vi "TDMS Read Channel Custom Fields.vi"(4 "MN":string, 5 "System or ALL Combined Fields":T1[](array[typedef]), 6 "SN":string, 7 "Group Name":string, 8 "error in (no error)":errorcluster, 9 "Channel":string, 10 "Custom Field Records to Search":string[](array[string]), 11 "tdms file ref":refnum<k34>) -> (0 "error out":errorcluster, 2 "Custom Fields":T1[](array[typedef]), 3 "tdms file ref":refnum<k34>)   [LabVIEW 2011]
uses:
  typedefs/Field Record.ctl
  typedefs/Field DataTypes.ctl
  typedefs/Field NextItem.ctl
panel:
  out "x-y 2":u32
  out "x-y":u32
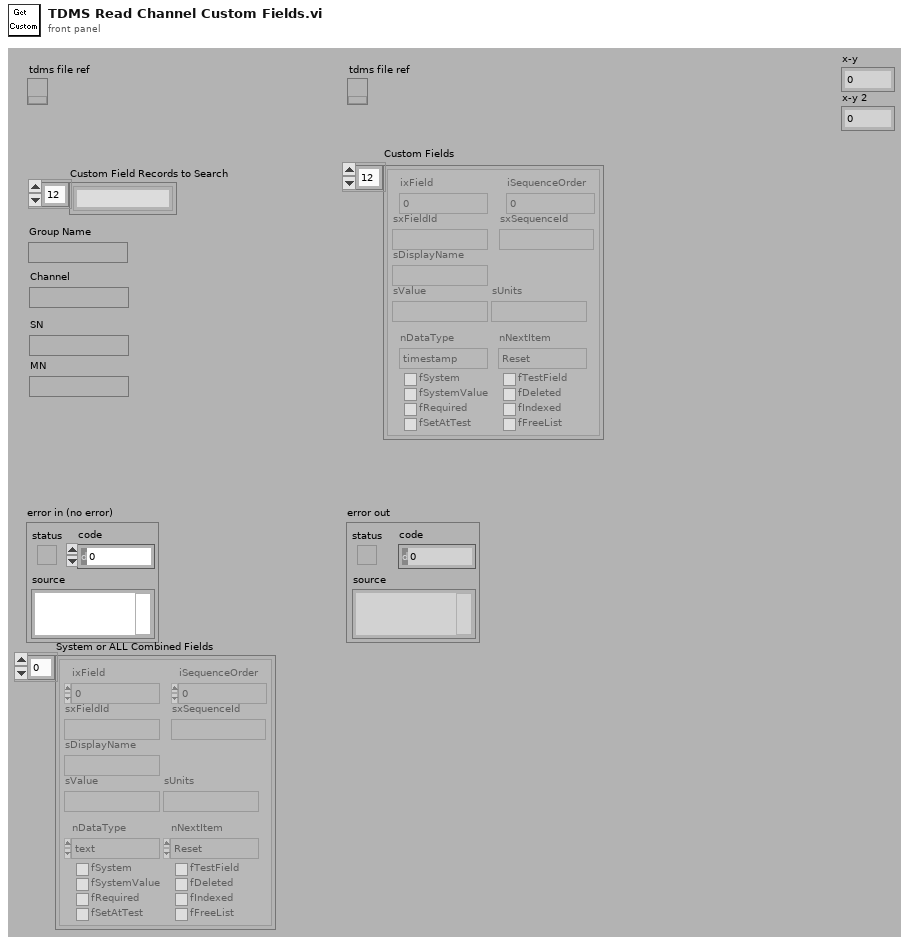
[diagram p1: front panel]
types:
  T1 = typedef "Field Record.ctl" = cluster{"ixField":i32, "iSequenceOrder":i32, "sxFieldId":string, "sxSequenceId":string, "sDisplayName":string, "sValue":string, "sUnits":string, "nDataType":T2, "nNextItem":T3, "fSystem":bool, "fSystemValue":bool, "fRequired":bool, "fSetAtTest":bool, "fTestField":bool, "fDeleted":bool, "fIndexed":bool, "fFreeList":bool}
  T2 = typedef "Field DataTypes.ctl" = enum32{"text", "numeric", "list", "timestamp", "boolean"}
  T3 = typedef "Field NextItem.ctl" = enum32{"Reset", "Retain", "Auto-Increment"}
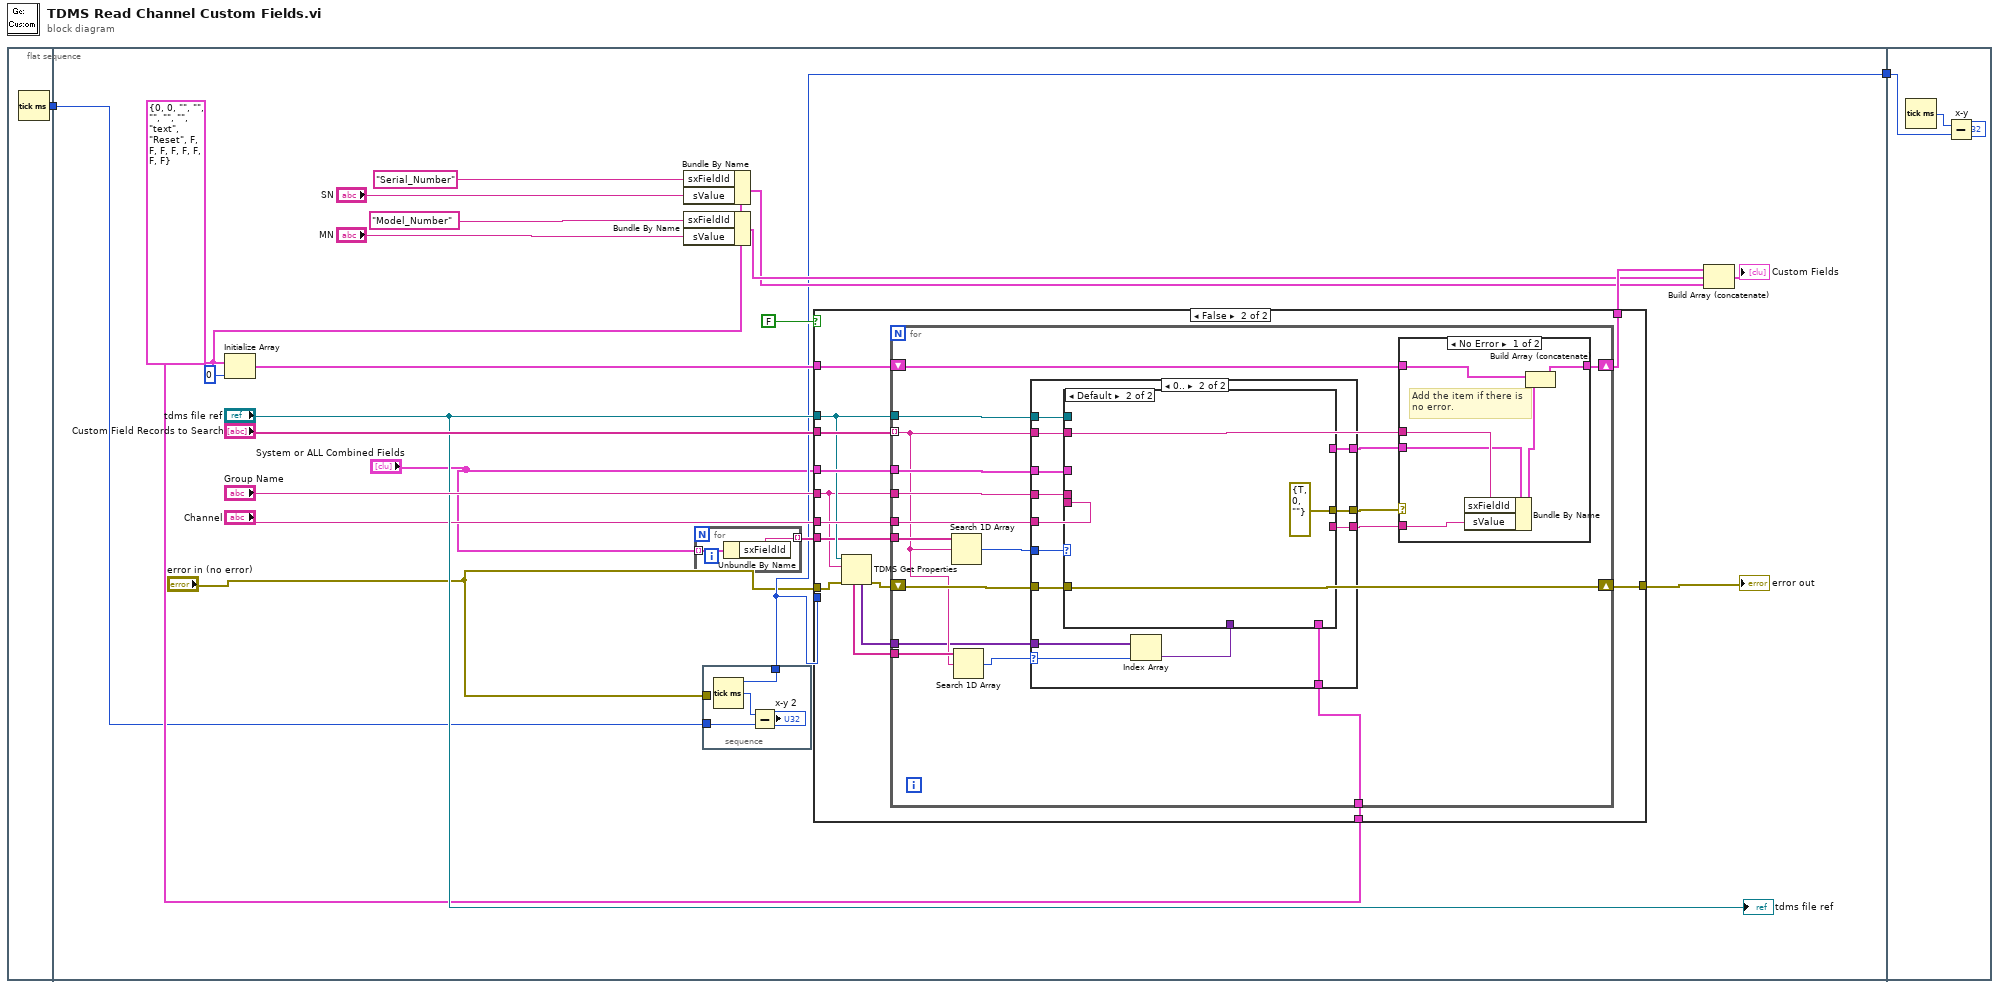
[diagram p0: block diagram]
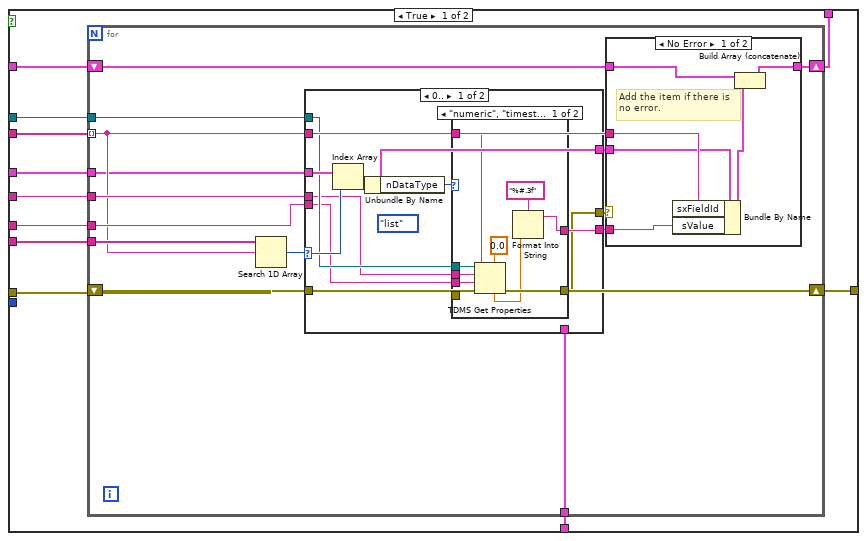
[diagram p2: hidden frame]
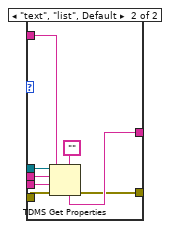
[diagram p3: hidden frame]
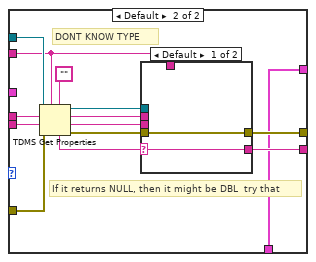
[diagram p4: hidden frame]
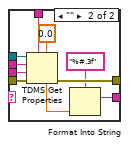
[diagram p5: hidden frame]
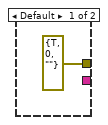
[diagram p7: hidden frame]
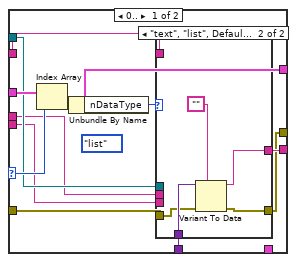
[diagram p8: hidden frame]
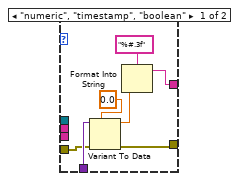
[diagram p9: hidden frame]
diagram:
  n1 = flat-sequence {
    tunnel: [w3] -> w1
    tunnel: [w7] -> w2
    tunnel: w1 -> [w6]
    tunnel: w2 -> [w197]
    frame #0 {
      n2 = Tick Count (ms)() -> (millisecond timer value=w3:u32)
    }
    frame #1 {
      w17 = T1 {"ixField"=0, "iSequenceOrder"=0, "sxFieldId"="", "sxSequenceId"="", "sDisplayName"="", "sValue"="", "sUnits"="", "nDataType"=enum."text", "nNextItem"=enum."Reset", "fSystem"=FALSE, "fSystemValue"=FALSE, "fRequired"=FALSE, "fSetAtTest"=FALSE, "fTestField"=FALSE, "fDeleted"=FALSE, "fIndexed"=FALSE, "fFreeList"=FALSE} ("Field Record")
      n3 = Initialize Array(w17, 0 ("dimension size")) -> (w25:T1[])
      n4 = Bundle By Name(cluster=w17, "sxFieldId"="Serial_Number", "sValue"="SN") -> (w9:T1)
      n5 = Bundle By Name(cluster=w17, "sxFieldId"="Model_Number", "sValue"="MN") -> (w10:T1)
      n6 = for {
        tunnel: "System or ALL Combined Fields" -> [w195] mode=indexing
        tunnel: [w194] -> w18 mode=indexing
        n7 = Unbundle By Name(w195) -> ("sxFieldId"=w194:string)
      }
      n8 = stacked-sequence {
        tunnel: "error in (no error)" -> [_]
        tunnel: [w28] -> w7
        tunnel: w6 -> [w27]
        frame #0 {
          n9 = Tick Count (ms)() -> (millisecond timer value=w28:u32)
          n10 = Subtract(x=w28, y=w27) -> (x-y=→"x-y 2":u32)
        }
      }
      n11 = case shown="False" FALSE {
        tunnel: w25 -> [w39 w129]
        tunnel: [w38 w128] -> w23
        tunnel: "Custom Field Records to Search" -> [w37 w127]
        tunnel: "Group Name" -> [w36 w118]
        tunnel: "tdms file ref" -> [w35 w120]
        tunnel: "Channel" -> [w34 w126]
        tunnel: "error in (no error)" -> [w33 w122]
        tunnel: w18 -> [w32 w119]
        tunnel: "System or ALL Combined Fields" -> [w31 w125]
        tunnel: w17 -> [w30 w124]
        tunnel: [w29 w123] -> w11
        tunnel: w7 -> [_ _]
        frame True {
          n12 = for {
            shift-right: [w51] -> w38
            shift-left: w33 -> [w51]
            shift-right: [w52] -> w29
            shift-left: w39 -> [w53]
            tunnel: w35 -> [w48]
            tunnel: w37 -> [w44] mode=indexing
            tunnel: w36 -> [w49]
            tunnel: w30 -> [w40]
            tunnel: w34 -> [w46]
            tunnel: w32 -> [w45]
            tunnel: w31 -> [w42]
            n13 = Search 1D Array(1D array=w45, element=w44) -> (index of element=w43:i32)  [unwired: 1 out]
            n14 = case shown="0.." w43 {
              selector: w43 -> [w63 _]
              tunnel: w51 -> [w62 w96]
              tunnel: [w56 w95] -> w50
              tunnel: w49 -> [w60 w94]
              tunnel: w48 -> [w61 w93]
              tunnel: [w55 w92] -> w47
              tunnel: w46 -> [w59 w91]
              tunnel: w44 -> [w57 w84]
              tunnel: w42 -> [w64 _]
              tunnel: [w54 w83] -> w41
              tunnel: w40 -> [_ w83]
              frame 0.. {
                (unwired) Field_DataTypes."list" ("nDataType")
                n15 = Index Array(array=w64, index=w63) -> (element=w54:T1)
                n16 = Unbundle By Name(w54) -> ("nDataType"=w58:T2)
                n17 = case shown="\"numeric\", \"timestamp\", \"boolean\"" w58 {
                  tunnel: w62 -> [w74 w82]
                  tunnel: w61 -> [w73 w81]
                  tunnel: w60 -> [w72 w80]
                  tunnel: w59 -> [w71 w79]
                  tunnel: w57 -> [w69 w78]
                  tunnel: [w67 w76] -> w56
                  tunnel: [w66 w75] -> w55
                  frame "numeric", "timestamp", "boolean" {
                    n18 = TDMS Get Properties(5:0.0, 7:w69, 8:w74, 9:w71, 10:w72, 11:w73) -> (0:w66:errorcluster, 4:w68:dbl)  [unwired: 4 out]
                    n19 = Format Into String(format string="%#.3f", w68) -> (resulting string=w67:string)  [unwired: 2 in, 1 out]
                  }
                  frame "text", "list", Default {
                    n20 = TDMS Get Properties(5:"", 7:w78, 8:w82, 9:w79, 10:w80, 11:w81) -> (0:w75:errorcluster, 4:w76:string)  [unwired: 4 out]
                  }
                }
              }
              frame Default {
                # "DONT KNOW TYPE"
                # "If it returns NULL, then it might be DBL  try that"
                n21 = TDMS Get Properties(5:"", 7:w84, 8:w96, 9:w91, 10:w94, 11:w93) -> (0:w89:errorcluster, 1:w85:string, 2:w86:string, 3:w88:refnum<k34>, 4:w87:string)  [unwired: 1 out]
                n22 = case shown="Default" w87 {
                  selector: w87 -> [w97 _]
                  tunnel: w89 -> [w98 w108]
                  tunnel: w88 -> [_ w107]
                  tunnel: w84 -> [_ w106]
                  tunnel: [w98 w105] -> w92
                  tunnel: [w97 w102] -> w95
                  tunnel: w86 -> [_ w101]
                  tunnel: w85 -> [_ w100]
                  frame Default {
                  }
                  frame "" {
                    n23 = TDMS Get Properties(5:0.0, 7:w106, 8:w108, 9:w100, 10:w101, 11:w107) -> (0:w105:errorcluster, 4:w104:dbl)  [unwired: 4 out]
                    n24 = Format Into String(format string="%#.3f", w104) -> (resulting string=w102:string)  [unwired: 2 in, 1 out]
                  }
                }
              }
            }
            n25 = case shown="No Error" w47 {
              tunnel: w53 -> [w114 w115]
              tunnel: [w113 w115] -> w52
              tunnel: w50 -> [w111 _]
              tunnel: w44 -> [w110 _]
              tunnel: w41 -> [w109 _]
              frame No Error {
                # "Add the item if there is\nno error."
                n26 = Bundle By Name(cluster=w109, "sxFieldId"=w110, "sValue"=w111) -> (w112:T1)
                n27 = Build Array (concatenate)(w114, w112) -> (w113:T1[])
              }
              frame Error {
              }
            }
          }
        }
        frame False {
          n28 = TDMS Get Properties(8:w122, 10:w118, 11:w120) -> (0:w121:errorcluster, 4:w116:variant[], 6:w117:string[])  [unwired: 3 in, 3 out]
          n29 = for {
            shift-right: [w144] -> w128
            shift-left: w121 -> [w144]
            shift-right: [w145] -> w123
            shift-left: w129 -> [w146]
            tunnel: w120 -> [w141]
            tunnel: w127 -> [w132] mode=indexing
            tunnel: w118 -> [w142]
            tunnel: w124 -> [w135]
            tunnel: w126 -> [w139]
            tunnel: w119 -> [w134]
            tunnel: w125 -> [w137]
            tunnel: w117 -> [w133]
            tunnel: w116 -> [w130]
            n30 = Search 1D Array(1D array=w134, element=w132) -> (index of element=w138:i32)  [unwired: 1 out]
            n31 = Search 1D Array(1D array=w133, element=w132) -> (index of element=w131:i32)  [unwired: 1 out]
            n32 = case shown="0.." w131 {
              selector: w131 -> [_ w149]
              tunnel: w144 -> [_ w161]
              tunnel: [_ w160] -> w143
              tunnel: w142 -> [_ w159]
              tunnel: w141 -> [_ w158]
              tunnel: [errorcluster {"status"=TRUE, "code"=0, "source"=""} ("error out") w157] -> w140
              tunnel: w139 -> [_ w156]
              tunnel: w138 -> [_ w155]
              tunnel: w137 -> [_ w154]
              tunnel: [_ w153] -> w136
              tunnel: w135 -> [_ w152]
              tunnel: w132 -> [_ w151]
              tunnel: w130 -> [_ w150]
              frame Default {
              }
              frame 0.. {
                n33 = Index Array(array=w150, index=w149) -> (element=w148:variant)
                n34 = case shown="Default" w155 {
                  selector: w155 -> [w172 _]
                  tunnel: w161 -> [w171 _]
                  tunnel: [w165 _] -> w160
                  tunnel: w159 -> [w169 _]
                  tunnel: w158 -> [w170 _]
                  tunnel: [w164 errorcluster {"status"=TRUE, "code"=0, "source"=""} ("error out")] -> w157
                  tunnel: w156 -> [w168 _]
                  tunnel: w151 -> [w166 _]
                  tunnel: w154 -> [w173 _]
                  tunnel: [w163 _] -> w153
                  tunnel: w152 -> [_ _]
                  tunnel: w148 -> [w162 _]
                  frame 0.. {
                    (unwired) Field_DataTypes."list" ("nDataType")
                    n35 = Index Array(array=w173, index=w172) -> (element=w163:T1)
                    n36 = Unbundle By Name(w163) -> ("nDataType"=w167:T2)
                    n37 = case shown="\"text\", \"list\", Default" w167 {
                      tunnel: w171 -> [w176 w183]
                      tunnel: w170 -> [_ _]
                      tunnel: w169 -> [_ _]
                      tunnel: w168 -> [_ _]
                      tunnel: w166 -> [_ _]
                      tunnel: [w180 w181] -> w165
                      tunnel: [w174 w182] -> w164
                      tunnel: w162 -> [w177 w184]
                      frame "numeric", "timestamp", "boolean" {
                        n38 = Variant To Data(error in=w176, type=0.0, Variant=w177) -> (data=w175:dbl, error out=w174:errorcluster)
                        n39 = Format Into String(format string="%#.3f", w175) -> (resulting string=w180:string)  [unwired: 2 in, 1 out]
                      }
                      frame "text", "list", Default {
                        n40 = Variant To Data(error in=w183, type="", Variant=w184) -> (data=w181:string, error out=w182:errorcluster)
                      }
                    }
                  }
                  frame Default {
                  }
                }
              }
            }
            n41 = case shown="No Error" w140 {
              tunnel: w146 -> [w192 w193]
              tunnel: [w191 w193] -> w145
              tunnel: w143 -> [w189 _]
              tunnel: w132 -> [w188 _]
              tunnel: w136 -> [w187 _]
              frame No Error {
                # "Add the item if there is\nno error."
                n42 = Bundle By Name(cluster=w187, "sxFieldId"=w188, "sValue"=w189) -> (w190:T1)
                n43 = Build Array (concatenate)(w192, w190) -> (w191:T1[])
              }
              frame Error {
              }
            }
          }
        }
      }
      "error out" <- w23
      n44 = Build Array (concatenate)(w11, w10, w9) -> (→"Custom Fields":T1[])
      "tdms file ref" <- "tdms file ref"
    }
    frame #2 {
      n45 = Tick Count (ms)() -> (millisecond timer value=w198:u32)
      n46 = Subtract(x=w198, y=w197) -> (x-y=→"x-y":u32)
    }
  }
